vi "FTW-TransferClient-S3-TransferUtility-Get.vi"(0 "Transfer Client":refnum<class "FTW-TransferClient-S3.lvclass">, 11 "error in":errorcluster) -> (4 "Transfer Client out":refnum<class "FTW-TransferClient-S3.lvclass">, 6 "Transfer Utility ref":refnum<k24>, 15 "error out":errorcluster)   [LabVIEW 2013, in "FTW-TransferClient-S3.lvclass"]
uses:
  FTW-TransferClient-S3.lvclass
  C:/Jobs/Tools/featherweight-trunk/Windows/src/Transfer Client/S3/AWSSDK.dll
  AWSSDK.dll
  FTW-TransferClient-S3.lvclass/FTW-TransferClient-S3.ctl
panel:
  # "Inputs"
  # "Outputs"
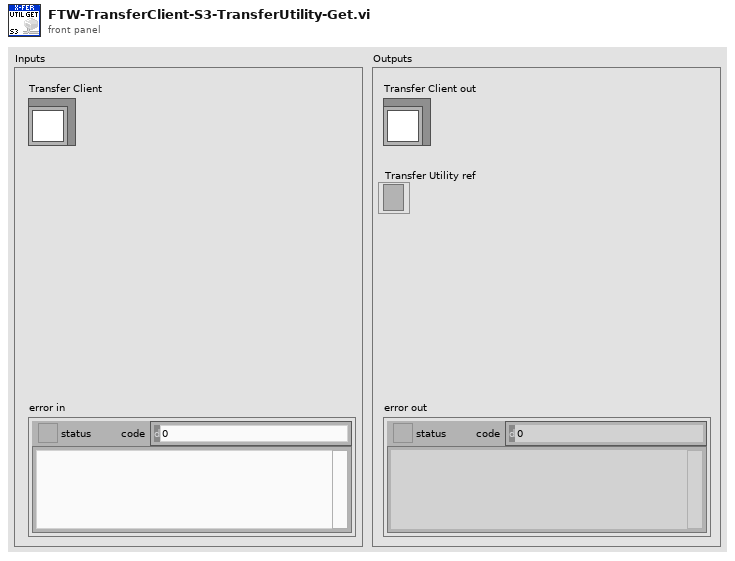
[diagram p1: front panel]
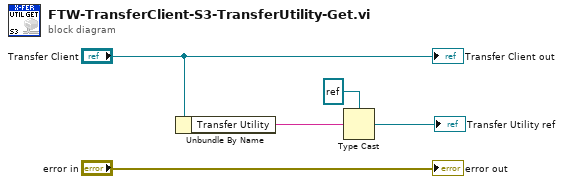
[diagram p0: block diagram]
diagram:
  n1 = Unbundle By Name("Transfer Client") -> ("Transfer Utility"=w4:string)
  n2 = Type Cast(type=refnum<k24> refnum ("Transfer Utility ref"), x=w4) -> (*(type *) &x=→"Transfer Utility ref":refnum<k24>)
  "error out" <- "error in"
  "Transfer Client out" <- "Transfer Client"
